vi "Get AI Channel Name.vi"(6 "AI Channel Names":string[](array[string])=["A/AI0", "A/AI1", "A/AI2", "A/AI3", "B/AI0", "B/AI1", "B/AI2", "B/AI3", "C/AI0", "C/AI1"], 7 "Error In":errorcluster, 9 "AI Channel Nums":u8[](array[numeric])) -> (0 "Error Out":errorcluster, 2 "AI Channels":string[](array[string]))   [LabVIEW 2020, in "LMH-LINX.lvlib" / "myRIO.lvlib"]
doc: "Get AI channel names (strings) from channel numbers."
uses:
  myRIO.lvlib
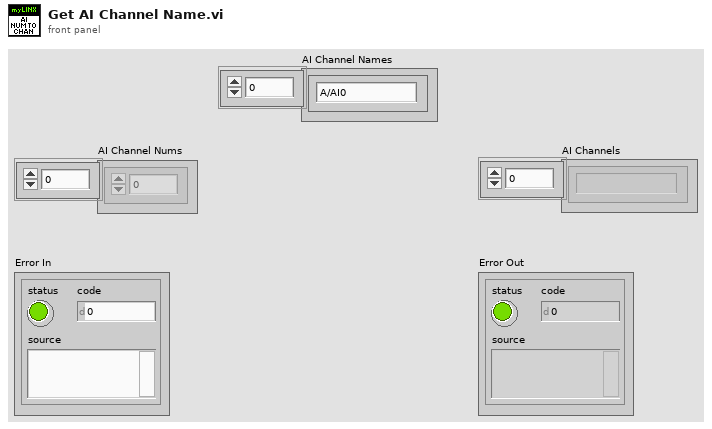
[diagram p1: front panel]
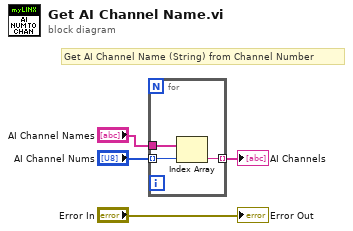
[diagram p0: block diagram]
diagram:
  # "Get AI Channel Name (String) from Channel Number"
  n1 = for {
    tunnel: "AI Channel Names" -> [w7]
    tunnel: "AI Channel Nums" -> [w6] mode=indexing
    tunnel: [w5] -> w3 mode=indexing
    n2 = Index Array(array=w7, index=w6) -> (element=w5:string)
  }
  "AI Channels" <- w3
  "Error Out" <- "Error In"
